vi "HFRR ADV v020 new software.vi"() -> ()   [LabVIEW 2025] (continued)
        n903 = call "File Dialog"("start path"=path "C:/LAB-IQ/images", "error in"=w1078) -> ("selected path"=w1067:path, "error out"=w1076:errorcluster)  [unwired: 10 in, 2 out]
        "Image path  2" <- w1067
        n904 = call <vilib>:"Clear Errors.vi"("error in (no error)"=w1076) -> ("error out"=w1075:errorcluster)  [unwired: 5 in, 1 out]
        n905 = call "IMAGE ANALYSIS.vi"("Enum"=POST_ANALYSIS_ENUM."OPEN FILE", "error in"=w1075, "File Path"=w1067) -> ("error out"=w1074:errorcluster)  [unwired: 7 in, 1 out]
        n906 = call <vilib>:"Clear Errors.vi"("error in (no error)"=w1074) -> ("error out"=w1073:errorcluster)  [unwired: 5 in, 1 out]
        n907 = call "IMAGE ANALYSIS.vi"("Enum"=POST_ANALYSIS_ENUM."SHOW UI", "error in"=w1073) -> ("error out"=w1071:errorcluster)  [unwired: 8 in, 1 out]
        n908 = local write "Zoom Factore"(100.0 ("Zoom Factore")) -> ()
      }
    }
    n909 = case shown="True" w762 {
      selector: w762 -> [_ w1050]
      tunnel: w754 -> [w1047 w1055]
      tunnel: [w1047 w1049] -> _
      frame False {
      }
      frame True {
        n910 = Not(x=w1050) -> (.not. x?=w1048:bool)
        n911 = local read "Zoom Factore"() -> (w1053:dbl)
        n912 = local write "OUT"(w1048) -> ()
        n913 = call "IMAGE ANALYSIS.vi"("Enum"=POST_ANALYSIS_ENUM."ZOOM OUT", "error in"=w1055) -> ("error out"=w1049:errorcluster)  [unwired: 8 in, 1 out]
        n914 = Divide(x=w1053, y=1.2) -> (x/y=w1051:dbl)
        n915 = local write "Zoom Factore"(w1051) -> ()
      }
    }
    n916 = case shown="True" w763 {
      selector: w763 -> [_ w1059]
      tunnel: w754 -> [w1056 w1064]
      tunnel: [w1056 w1057] -> _
      frame False {
      }
      frame True {
        n917 = Not(x=w1059) -> (.not. x?=w1058:bool)
        n918 = local read "Zoom Factore"() -> (w1062:dbl)
        n919 = local write "In"(w1058) -> ()
        n920 = call "IMAGE ANALYSIS.vi"("Enum"=POST_ANALYSIS_ENUM."ZOOM IN", "error in"=w1064) -> ("error out"=w1057:errorcluster)  [unwired: 8 in, 1 out]
        n921 = Multiply(x=w1062, y=1.2) -> (x*y=w1060:dbl)
        n922 = local write "Zoom Factore"(w1060) -> ()
      }
    }
    n923 = case shown="True" w759 {
      selector: w759 -> [_ w1031]
      tunnel: w754 -> [w1029 w1033]
      tunnel: [w1029 w1032] -> _
      frame False {
      }
      frame True {
        n924 = Not(x=w1031) -> (.not. x?=w1030:bool)
        n925 = local write "Clear ROI Tool"(w1030) -> ()
        n926 = call "IMAGE ANALYSIS.vi"("Enum"=POST_ANALYSIS_ENUM."CLEAR ROI", "error in"=w1033) -> ("error out"=w1032:errorcluster)  [unwired: 8 in, 1 out]
      }
    }
    n927 = case shown="True" w761 {
      selector: w761 -> [_ w1043]
      tunnel: w754 -> [w1041 w1046]
      tunnel: [w1041 w1044] -> _
      frame False {
      }
      frame True {
        n928 = Not(x=w1043) -> (.not. x?=w1042:bool)
        n929 = local write "line tool"(w1042) -> ()
        n930 = call "IMAGE ANALYSIS.vi"("Enum"=POST_ANALYSIS_ENUM."DRAW LINE", "error in"=w1046) -> ("error out"=w1044:errorcluster)  [unwired: 8 in, 1 out]
      }
    }
    n931 = case shown="True" w760 {
      selector: w760 -> [_ w1037]
      tunnel: w754 -> [w1035 w1039]
      tunnel: [w1035 w1038] -> _
      frame False {
      }
      frame True {
        n932 = Not(x=w1037) -> (.not. x?=w1036:bool)
        n933 = local write "Rectangle Tool"(w1036) -> ()
        n934 = call "IMAGE ANALYSIS.vi"("Enum"=POST_ANALYSIS_ENUM."DRAW REC", "error in"=w1039) -> ("error out"=w1038:errorcluster)  [unwired: 8 in, 1 out]
      }
    }
    n935 = local read "SCAR MEASURMENT"() -> (w747:enum32{"Auto Scar", "Manual Scar"})
    n936 = local read "Fit to Screen Tool"() -> (w756:bool)
    n937 = local read "Resize Tool"() -> (w755:bool)
    n938 = case shown="\"Manual Scar\", Default" w747 {
      frame "Auto Scar" {
        n939 = property on="Cap Live Image" class="Bool (strict)"("BoolText.Text"="Report" ("Boolean Text.Text")) -> ()  [unwired: 2 in, 2 out]
      }
      frame "Manual Scar", Default {
        n940 = property on="Cap Live Image" class="Bool (strict)"("BoolText.Text"="Save Image" ("Boolean Text.Text")) -> ()  [unwired: 2 in, 2 out]
      }
    }
    n941 = local read "ROI Color Tool"() -> (w757:bool)
    n942 = local read "Pan Tool"() -> (w758:bool)
    n943 = case shown="True" w758 {
      selector: w758 -> [_ w1025]
      tunnel: w754 -> [w1023 w1027]
      tunnel: [w1023 w1026] -> _
      frame False {
      }
      frame True {
        n944 = Not(x=w1025) -> (.not. x?=w1024:bool)
        n945 = call "IMAGE ANALYSIS.vi"("Enum"=POST_ANALYSIS_ENUM."PAN", "error in"=w1027) -> ("error out"=w1026:errorcluster)  [unwired: 8 in, 1 out]
        n946 = local write "Pan Tool"(w1024) -> ()
      }
    }
    n947 = case shown="True" w755 {
      selector: w755 -> [_ w1009]
      tunnel: w754 -> [w1004 w1006]
      tunnel: [w1004 w1005] -> _
      frame False {
      }
      frame True {
        n948 = Not(x=w1009) -> (.not. x?=w1008:bool)
        n949 = local write "Resize Tool"(w1008) -> ()
        n950 = call "IMAGE ANALYSIS.vi"("Enum"=POST_ANALYSIS_ENUM."RESIZE MODE", "error in"=w1006) -> ("error out"=w1005:errorcluster)  [unwired: 8 in, 1 out]
      }
    }
    n951 = case shown="True" w756 {
      selector: w756 -> [_ w1014]
      tunnel: [w1010 w1015] -> _
      tunnel: w754 -> [w1010 w1013]
      frame False {
      }
      frame True {
        n952 = Not(x=w1014) -> (.not. x?=w1012:bool)
        n953 = local write "Zoom Factore"(100.0 ("Zoom Factore")) -> ()
        n954 = local write "Fit to Screen Tool"(w1012) -> ()
        n955 = call "IMAGE ANALYSIS.vi"("Enum"=POST_ANALYSIS_ENUM."FIT", "error in"=w1013) -> ("error out"=w1015:errorcluster)  [unwired: 8 in, 1 out]
      }
    }
    n956 = case shown="True" w757 {
      selector: w757 -> [_ w1020]
      tunnel: [w1017 w1021] -> _
      tunnel: w754 -> [w1017 w1018]
      frame False {
      }
      frame True {
        n957 = Not(x=w1020) -> (.not. x?=w1019:bool)
        n958 = local write "ROI Color Tool"(w1019) -> ()
        n959 = call "IMAGE ANALYSIS.vi"("Enum"=POST_ANALYSIS_ENUM."SET ROI COLOR", "error in"=w1018) -> ("error out"=w1021:errorcluster)  [unwired: 8 in, 1 out]
      }
    }
    n960 = local read "Quit"() -> (w771:bool)
  }
  n961 = while {
    stop <- w1105 stop-if-true
    n962 = local read "Image Path"() -> (w1108:path)
    n963 = local read "Print 3"() -> (w1111:bool)
    n964 = Equal?(x=w1108, y=path "") -> (x = y?=w1107:bool)
    n965 = Not(x=w1107) -> (.not. x?=w1106:bool)
    n966 = property on="Print 3" class="Bool (strict)"("Visible"=w1106) -> ()  [unwired: 2 in, 2 out]
    n967 = case shown="True" w1111 {
      frame False {
        n968 = local write "Rd"(TRUE ("Boolean 7")) -> ()
      }
      frame True {
        n969 = flat-sequence {
          tunnel: [w1151] -> w1119
          tunnel: [w1138] -> w1117
          tunnel: [w1148] -> w1113
          tunnel: w1119 -> [w1160]
          tunnel: [w1160] -> w1118
          tunnel: w1117 -> [w1159]
          tunnel: [w1159] -> w1116
          tunnel: [w1157] -> w1115
          tunnel: [w1156] -> w1114
          tunnel: w1113 -> [w1156]
          tunnel: w1118 -> [w1162]
          tunnel: w1116 -> [w1163]
          tunnel: w1115 -> [_]
          tunnel: w1114 -> [w1161]
          frame #0 {
            n970 = case shown="True" "Rd" {
              frame False {
              }
              frame True {
                n971 = while {
                  tunnel: "abcdefABCDEF" ("string 2") -> [w1130]
                  shift-right: [w1128] -> w1122
                  shift-left: "" -> [w1127]
                  i -> [w1137]
                  stop <- w1136 stop-if-true
                  n972 = Random Number (0-1)() -> (number: 0 to 1=w1131:dbl)
                  n973 = Multiply(x=w1131, y=62.0) -> (x*y=w1133:dbl)
                  n974 = Decrement(x="Length 2") -> (x-1=w1126:i16)
                  n975 = To Word Integer(number=w1133) -> (16bit integer=w1134:i16)
                  n976 = String Subset(string=w1130, offset (0)=w1134, length (rest)=1 ("length (rest)")) -> (substring=w1129:string)
                  n977 = Greater Or Equal?(x=w1137, y=w1126) -> (x >= y?=w1136:bool)
                  n978 = Concatenate Strings(w1129, w1127) -> (w1128:string)
                }
                "String 10" <- w1122
                n979 = local write "Rd"(FALSE ("Boolean 7")) -> ()
              }
            }
          }
          frame #1 {
            w1149 = "_resized.jpg" ("command line")
            (unwired) ".jpg -resize 320x240 " ("string")
            (unwired) "Choose an Image File" ("prompt")
            # "-resize 1798x425"
            n980 = local read "Image Path"() -> (w1143:path)
            n981 = Strip Path(path=w1143) -> (stripped path=w1138:path, name=w1139:string)
            n982 = Match Pattern(string=w1139, regular expression=".jpg") -> (before substring=→"before substring 2":string, after substring=→"after substring":string)  [unwired: 1 in, 2 out]
            n983 = Match Pattern(string=w1139, regular expression="\\") -> (before substring=w1145:string)  [unwired: 1 in, 3 out]
            n984 = Match Pattern(string=w1145, regular expression=".jpg") -> (before substring=w1144:string)  [unwired: 1 in, 3 out]
            n985 = Concatenate Strings("cmd /c convert " ("string"), w1144, ".jpg -resize 320x240  " ("command line"), w1144, w1149) -> (w1152:string)
            n986 = call <vilib>:"System Exec.vi"("run minimized? (F)"=TRUE, "wait until completion? (T)"=TRUE, "working directory"=w1138, "command line"=w1152) -> ("error out"=w1151:errorcluster)  [unwired: 4 in, 3 out]
            "error out 2" <- w1151
            n987 = Concatenate Strings(w1144, w1149) -> (w1148:string)
          }
          frame #2 {
            n988 = Wait (ms)(milliseconds to wait=u32 2000 ("millisecond timer value")) -> (millisecond timer value=w1157:u32)
          }
          frame #3 {
            n989 = case shown="No Error" w1162 {
              tunnel: w1163 -> [w1166 _]
              tunnel: w1161 -> [w1164 _]
              frame No Error {
                (unwired) ".jpg" ("string")
                n990 = Path To String(path=w1166) -> (string=w1170:string)
                n991 = Concatenate Strings(w1170, "\\" ("string"), w1164) -> (w1169:string)
                n992 = String To Path(string=w1169) -> (path=w1168:path)
                n993 = call <vilib>:"Read JPEG File.vi"("path to JPEG file"=w1168) -> ("image data"=w1172:T16)  [unwired: 8 in, 2 out]
                "image data" <- w1172
                n994 = local write "Print 3"(FALSE ("Print 2")) -> ()
                n995 = call <vilib>:"Draw Flattened Pixmap.vi"("image data"=w1172) -> ("new picture"=→"new picture":picture)  [unwired: 8 in]
              }
              frame Error {
              }
            }
          }
        }
      }
    }
    n996 = Wait (ms)(milliseconds to wait=u32 20 ("millisecond timer value")) -> ()  [unwired: 1 out]
    n997 = local read "Quit"() -> (w1105:bool)
  }
  n998 = while {
    tunnel: w39 -> [_]
    tunnel: w23 -> [_]
    stop <- w1203 stop-if-true
    # "New Adv Logics"
    n999 = local read "Main Tab"() -> (w1183:T2)
    n1000 = local read "Main Tab"() -> (w1201:T2)
    n1001 = local read "Sign In"() -> (w1200:bool)
    n1002 = case shown="\"Adv Scar\"" w1183 {
      frame "HOME", Default {
        n1003 = local read "LIVE FEED MIN TEMP"() -> (w1336:bool)
        n1004 = local write "LIVE FEED MAX TEMP"(TRUE ("LIVE FEED MAX TEMP")) -> ()
        n1005 = local read "CAMERA ROI MIN TEMP"() -> (w1334:bool)
        n1006 = case shown="True" w1336 {
          selector: w1336 -> [_ w1343]
          frame False {
          }
          frame True {
            n1007 = Not(x=w1343) -> (.not. x?=w1342:bool)
            n1008 = local write "LIVE FEED MIN TEMP"(w1342) -> ()
            n1009 = call "CAMERA LIVE FEED FGV.vi"("Enum - Menu"=CAMERA_LIVE_FEED_ENUM."CAMERA MINIMIZE") -> ()  [unwired: 9 in, 2 out]
          }
        }
        n1010 = case shown="True" w1334 {
          selector: w1334 -> [_ w1340]
          frame False {
          }
          frame True {
            n1011 = Not(x=w1340) -> (.not. x?=w1339:bool)
            n1012 = local write "CAMERA ROI MIN TEMP"(w1339) -> ()
            n1013 = call "IMAGE ANALYSIS.vi"("Enum"=POST_ANALYSIS_ENUM."MINIMIZE UI") -> ()  [unwired: 9 in, 2 out]
          }
        }
        n1014 = local write "CAMERA ROI MAX TEMP"(TRUE ("CAMERA ROI MAX TEMP")) -> ()
      }
      frame "Test Setup" {
        n1015 = local read "LIVE FEED MIN TEMP"() -> (w1346:bool)
        n1016 = local read "CAMERA ROI MIN TEMP"() -> (w1344:bool)
        n1017 = local write "LIVE FEED MAX TEMP"(TRUE ("LIVE FEED MAX TEMP")) -> ()
        n1018 = case shown="True" w1346 {
          selector: w1346 -> [_ w1353]
          frame False {
          }
          frame True {
            n1019 = Not(x=w1353) -> (.not. x?=w1352:bool)
            n1020 = local write "LIVE FEED MIN TEMP"(w1352) -> ()
            n1021 = call "CAMERA LIVE FEED FGV.vi"("Enum - Menu"=CAMERA_LIVE_FEED_ENUM."CAMERA MINIMIZE") -> ()  [unwired: 9 in, 2 out]
          }
        }
        n1022 = case shown="True" w1344 {
          selector: w1344 -> [_ w1350]
          frame False {
          }
          frame True {
            n1023 = Not(x=w1350) -> (.not. x?=w1349:bool)
            n1024 = local write "CAMERA ROI MIN TEMP"(w1349) -> ()
            n1025 = call "IMAGE ANALYSIS.vi"("Enum"=POST_ANALYSIS_ENUM."MINIMIZE UI") -> ()  [unwired: 9 in, 2 out]
          }
        }
        n1026 = local write "CAMERA ROI MAX TEMP"(TRUE ("CAMERA ROI MAX TEMP")) -> ()
      }
      frame "Acquire" {
        n1027 = local read "LIVE FEED MIN TEMP"() -> (w1356:bool)
        n1028 = local write "LIVE FEED MAX TEMP"(TRUE ("LIVE FEED MAX TEMP")) -> ()
        n1029 = local read "CAMERA ROI MIN TEMP"() -> (w1354:bool)
        n1030 = case shown="True" w1356 {
          selector: w1356 -> [_ w1363]
          frame False {
          }
          frame True {
            n1031 = Not(x=w1363) -> (.not. x?=w1362:bool)
            n1032 = local write "LIVE FEED MIN TEMP"(w1362) -> ()
            n1033 = call "CAMERA LIVE FEED FGV.vi"("Enum - Menu"=CAMERA_LIVE_FEED_ENUM."CAMERA MINIMIZE") -> ()  [unwired: 9 in, 2 out]
          }
        }
        n1034 = case shown="True" w1354 {
          selector: w1354 -> [_ w1360]
          frame False {
          }
          frame True {
            n1035 = Not(x=w1360) -> (.not. x?=w1359:bool)
            n1036 = local write "CAMERA ROI MIN TEMP"(w1359) -> ()
            n1037 = call "IMAGE ANALYSIS.vi"("Enum"=POST_ANALYSIS_ENUM."MINIMIZE UI") -> ()  [unwired: 9 in, 2 out]
          }
        }
        n1038 = local write "CAMERA ROI MAX TEMP"(TRUE ("CAMERA ROI MAX TEMP")) -> ()
      }
      frame "Adv Scar" {
        n1039 = local read "CAMERA ROI MIN TEMP"() -> (w1364:bool)
        n1040 = case shown="True" "LIVE FEED MAX TEMP" {
          selector: "LIVE FEED MAX TEMP" -> [_ w1385]
          frame False {
          }
          frame True {
            n1041 = Not(x=w1385) -> (.not. x?=w1384:bool)
            n1042 = local write "LIVE FEED MAX TEMP"(w1384) -> ()
            n1043 = call "CAMERA LIVE FEED FGV.vi"("Enum - Menu"=CAMERA_LIVE_FEED_ENUM."CAMERA RESTORE") -> ("error out"=w1375:errorcluster)  [unwired: 9 in, 1 out]
            n1044 = Type Cast(type=30, x=0) -> (*(type *) &x=w1379:i32)
            n1045 = Add(x=w1379, y=48) -> (x+y=w1380:i32)
            n1046 = call "CAMERA LIVE FEED FGV.vi"("Enum - Menu"=CAMERA_LIVE_FEED_ENUM."CAMERA MODE SET", "error in (no error)"=w1375, "CAMERA MODE"=w1380) -> ("error out"=w1372:errorcluster)  [unwired: 7 in, 1 out]
            n1047 = call "CAMERA LIVE FEED FGV.vi"("Enum - Menu"=CAMERA_LIVE_FEED_ENUM."CAMERA GRAY", "error in (no error)"=w1372) -> ("error out"=w1371:errorcluster)  [unwired: 8 in, 1 out]
            n1048 = call "LIST FILE NAMES.vi"("error in (no error)"=w1371) -> ("error out"=w1381:errorcluster, "filenames"=w1382:string[])  [unwired: 9 in]
            n1049 = property on="FILE 3" class="CmbBox"(error in=w1381, "Strings[]"=w1382) -> ()  [unwired: 1 in, 2 out]
          }
        }
        n1050 = case shown="True" w1364 {
          selector: w1364 -> [_ w1370]
          frame False {
          }
          frame True {
            n1051 = Not(x=w1370) -> (.not. x?=w1369:bool)
            n1052 = local write "CAMERA ROI MIN TEMP"(w1369) -> ()
            n1053 = call "IMAGE ANALYSIS.vi"("Enum"=POST_ANALYSIS_ENUM."MINIMIZE UI") -> ()  [unwired: 9 in, 2 out]
          }
        }
        n1054 = local write "CAMERA ROI MAX TEMP"(TRUE ("CAMERA ROI MAX TEMP")) -> ()
        "LIVE FEED MIN TEMP" <- TRUE ("LIVE FEED MIN TEMP")
      }
      frame "Adv Scar Report" {
        n1055 = local read "CAMERA ROI MAX TEMP"() -> (w1386:bool)
        n1056 = local read "LIVE FEED MIN TEMP"() -> (w1388:bool)
        n1057 = local write "LIVE FEED MAX TEMP"(TRUE ("LIVE FEED MAX TEMP")) -> ()
        n1058 = case shown="True" w1388 {
          selector: w1388 -> [_ w1397]
          frame False {
          }
          frame True {
            n1059 = Not(x=w1397) -> (.not. x?=w1396:bool)
            n1060 = local write "LIVE FEED MIN TEMP"(w1396) -> ()
            n1061 = call "CAMERA LIVE FEED FGV.vi"("Enum - Menu"=CAMERA_LIVE_FEED_ENUM."CAMERA MINIMIZE") -> ()  [unwired: 9 in, 2 out]
          }
        }
        n1062 = case shown="True" w1386 {
          selector: w1386 -> [_ w1394]
          frame False {
          }
          frame True {
            n1063 = Not(x=w1394) -> (.not. x?=w1392:bool)
            n1064 = local write "CAMERA ROI MAX TEMP"(w1392) -> ()
            n1065 = call "IMAGE ANALYSIS.vi"("Enum"=POST_ANALYSIS_ENUM."SHOW UI") -> ("error out"=w1391:errorcluster)  [unwired: 9 in, 1 out]
            n1066 = call "LIST FILE NAMES.vi"("error in (no error)"=w1391) -> ("filenames"=w1390:string[])  [unwired: 9 in, 1 out]
            n1067 = property on="Test File List :" class="CmbBox"("Strings[]"=w1390) -> ()  [unwired: 2 in, 2 out]
          }
        }
        n1068 = local write "CAMERA ROI MIN TEMP"(TRUE ("CAMERA ROI MIN TEMP")) -> ()
      }
      frame "Compare Files" {
        n1069 = local read "LIVE FEED MIN TEMP"() -> (w1400:bool)
        n1070 = local write "LIVE FEED MAX TEMP"(TRUE ("LIVE FEED MAX TEMP")) -> ()
        n1071 = local read "CAMERA ROI MIN TEMP"() -> (w1398:bool)
        n1072 = case shown="True" w1400 {
          selector: w1400 -> [_ w1407]
          frame False {
          }
          frame True {
            n1073 = Not(x=w1407) -> (.not. x?=w1406:bool)
            n1074 = local write "LIVE FEED MIN TEMP"(w1406) -> ()
            n1075 = call "CAMERA LIVE FEED FGV.vi"("Enum - Menu"=CAMERA_LIVE_FEED_ENUM."CAMERA MINIMIZE") -> ()  [unwired: 9 in, 2 out]
          }
        }
        n1076 = case shown="True" w1398 {
          selector: w1398 -> [_ w1404]
          frame False {
          }
          frame True {
            n1077 = Not(x=w1404) -> (.not. x?=w1403:bool)
            n1078 = local write "CAMERA ROI MIN TEMP"(w1403) -> ()
            n1079 = call "IMAGE ANALYSIS.vi"("Enum"=POST_ANALYSIS_ENUM."MINIMIZE UI") -> ()  [unwired: 9 in, 2 out]
          }
        }
        n1080 = local write "CAMERA ROI MAX TEMP"(TRUE ("CAMERA ROI MAX TEMP")) -> ()
      }
      frame "About" {
        n1081 = local read "LIVE FEED MIN TEMP"() -> (w1410:bool)
        n1082 = local write "LIVE FEED MAX TEMP"(TRUE ("LIVE FEED MAX TEMP")) -> ()
        n1083 = local read "CAMERA ROI MIN TEMP"() -> (w1409:bool)
        n1084 = case shown="True" w1410 {
          selector: w1410 -> [_ w1417]
          frame False {
          }
          frame True {
            n1085 = Not(x=w1417) -> (.not. x?=w1416:bool)
            n1086 = local write "LIVE FEED MIN TEMP"(w1416) -> ()
            n1087 = call "CAMERA LIVE FEED FGV.vi"("Enum - Menu"=CAMERA_LIVE_FEED_ENUM."CAMERA MINIMIZE") -> ()  [unwired: 9 in, 2 out]
          }
        }
        n1088 = case shown="True" w1409 {
          selector: w1409 -> [_ w1414]
          frame False {
          }
          frame True {
            n1089 = Not(x=w1414) -> (.not. x?=w1413:bool)
            n1090 = local write "CAMERA ROI MIN TEMP"(w1413) -> ()
            n1091 = call "IMAGE ANALYSIS.vi"("Enum"=POST_ANALYSIS_ENUM."MINIMIZE UI") -> ()  [unwired: 9 in, 2 out]
          }
        }
        n1092 = local write "CAMERA ROI MAX TEMP"(TRUE ("CAMERA ROI MIN TEMP")) -> ()
      }
      frame "Advance" {
        n1093 = local read "LIVE FEED MIN TEMP"() -> (w1420:bool)
        n1094 = local write "LIVE FEED MAX TEMP"(TRUE ("LIVE FEED MAX TEMP")) -> ()
        n1095 = local read "CAMERA ROI MIN TEMP"() -> (w1418:bool)
        n1096 = case shown="True" w1420 {
          selector: w1420 -> [_ w1427]
          frame False {
          }
          frame True {
            n1097 = Not(x=w1427) -> (.not. x?=w1426:bool)
            n1098 = local write "LIVE FEED MIN TEMP"(w1426) -> ()
            n1099 = call "CAMERA LIVE FEED FGV.vi"("Enum - Menu"=CAMERA_LIVE_FEED_ENUM."CAMERA MINIMIZE") -> ()  [unwired: 9 in, 2 out]
          }
        }
        n1100 = local write "CAMERA ROI MAX TEMP"(TRUE ("CAMERA ROI MAX TEMP")) -> ()
        n1101 = case shown="True" w1418 {
          selector: w1418 -> [_ w1424]
          frame False {
          }
          frame True {
            n1102 = Not(x=w1424) -> (.not. x?=w1423:bool)
            n1103 = local write "CAMERA ROI MIN TEMP"(w1423) -> ()
            n1104 = call "IMAGE ANALYSIS.vi"("Enum"=POST_ANALYSIS_ENUM."MINIMIZE UI") -> ()  [unwired: 9 in, 2 out]
          }
        }
      }
      frame "Mooha" {
        n1105 = local read "LIVE FEED MIN TEMP"() -> (w1430:bool)
        n1106 = local write "LIVE FEED MAX TEMP"(TRUE ("LIVE FEED MAX TEMP")) -> ()
        n1107 = local read "CAMERA ROI MIN TEMP"() -> (w1428:bool)
        n1108 = case shown="True" w1430 {
          selector: w1430 -> [_ w1437]
          frame False {
          }
          frame True {
            n1109 = Not(x=w1437) -> (.not. x?=w1436:bool)
            n1110 = local write "LIVE FEED MIN TEMP"(w1436) -> ()
            n1111 = call "CAMERA LIVE FEED FGV.vi"("Enum - Menu"=CAMERA_LIVE_FEED_ENUM."CAMERA MINIMIZE") -> ()  [unwired: 9 in, 2 out]
          }
        }
        n1112 = local write "CAMERA ROI MAX TEMP"(TRUE ("CAMERA ROI MAX TEMP")) -> ()
        n1113 = case shown="True" w1428 {
          selector: w1428 -> [_ w1434]
          frame False {
          }
          frame True {
            n1114 = Not(x=w1434) -> (.not. x?=w1433:bool)
            n1115 = local write "CAMERA ROI MIN TEMP"(w1433) -> ()
            n1116 = call "IMAGE ANALYSIS.vi"("Enum"=POST_ANALYSIS_ENUM."MINIMIZE UI") -> ()  [unwired: 9 in, 2 out]
          }
        }
      }
    }
    n1117 = local read "Auto Start Test"() -> (w1174:bool)
    n1118 = case shown="True" "sign in temp" {
      frame False {
      }
      frame True {
        w1210 = 1 ("y")
        n1119 = local read "USERNAME"() -> (w1216:string)
        n1120 = local read "USER ID"() -> (w1213:string)
        n1121 = call <vilib>:"Trim Whitespace.vi"("string"=w1216) -> ("trimmed string"=w1215:string)  [unwired: 1 in]
        n1122 = call <vilib>:"Trim Whitespace.vi"("string"=w1213) -> ("trimmed string"=w1214:string)  [unwired: 1 in]
        n1123 = String Length(string=w1215) -> (length=w1212:i32)
        n1124 = String Length(string=w1214) -> (length=w1211:i32)
        n1125 = Greater?(x=w1212, y=w1210) -> (0:w1209:bool)
        n1126 = Greater?(x=w1211, y=w1210) -> (0:w1208:bool)
        n1127 = And(x=w1209, y=w1208) -> (x .and. y?=w1207:bool)
        n1128 = case shown="True" w1207 {
          frame False {
            n1129 = property on="Sign In" class="Bool (strict)"("DisabledEnum"=T19."Disabled" ("Disabled")) -> ()  [unwired: 2 in, 2 out]
          }
          frame True {
            n1130 = property on="Sign In" class="Bool (strict)"("DisabledEnum"=T19."Enabled" ("Disabled")) -> ()  [unwired: 2 in, 2 out]
          }
        }
      }
    }
    n1131 = local read "Air Temperature"() -> (w1191:bool)
    n1132 = local read "Coefficient Of Friction"() -> (w1192:bool)
    n1133 = case shown="False" w1174 {
      frame False {
        n1134 = local read "Auto stop temp"() -> (w1204:bool)
        n1135 = case shown="True" w1204 {
          frame False {
          }
          frame True {
            n1136 = local write "Auto Start Temp"(FALSE ("Auto Start Temp")) -> ()
          }
        }
      }
      frame True {
        "Auto stop temp" <- TRUE ("Auto stop temp")
      }
    }
    n1137 = local read "Humidity"() -> (w1190:bool)
    n1138 = case shown="\"HOME\"" w1201 {
      frame "HOME" {
        n1139 = local write "main tab sub"(enum32{"Page 1", "Page 2"}."Page 1" ("main tab sub")) -> ()
      }
      frame Default {
        n1140 = local write "main tab sub"(enum32{"Page 1", "Page 2"}."Page 2" ("main tab sub")) -> ()
      }
    }
    n1141 = case shown="True" w1200 {
      selector: w1200 -> [_ w1551]
      frame False {
      }
      frame True {
        n1142 = Not(x=w1551) -> (.not. x?=w1550:bool)
        n1143 = local write "Sign In"(w1550) -> ()
        n1144 = local write "Main Dashboard Buttons"(T24."Test Setup" ("Main Dashboard Buttons")) -> ()
      }
    }
    n1145 = case shown="\"Numeric Display\", Default" "Num/Graph" {
      frame "Numeric Display", Default {
        n1146 = property on="Single/Multiple" class="RadioBtnsControl (strict)"("Visible"=FALSE) -> ()  [unwired: 2 in, 2 out]
        n1147 = property on="Single - Graph" class="Ring (strict)"("Visible"=FALSE) -> ()  [unwired: 2 in, 2 out]
        n1148 = local write "Main Tab Display"(T4."Dashboard 1" ("Main Tab Display")) -> ()
      }
      frame "Graph Display" {
        n1149 = property on="Single/Multiple" class="RadioBtnsControl (strict)"("Visible"=TRUE) -> ()  [unwired: 2 in, 2 out]
        n1150 = case shown="\"Multiple\"" "Single/Multiple" {
          frame "Single ", Default {
            n1151 = property on="Single - Graph" class="Ring (strict)"("Visible"=TRUE) -> ()  [unwired: 2 in, 2 out]
            n1152 = local write "Main Tab Display"(T4."Dashboard 3" ("Main Tab Display")) -> ()
          }
          frame "Multiple" {
            n1153 = property on="Single - Graph" class="Ring (strict)"("Visible"=FALSE) -> ()  [unwired: 2 in, 2 out]
            n1154 = local write "Main Tab Display"(T4."Dashboard 2" ("Main Tab Display")) -> ()
          }
        }
      }
    }
    n1155 = local read "Stroke"() -> (w1189:bool)
    n1156 = local read "USERNAME"() -> (w1195:string)
    n1157 = local read "USER ID"() -> (w1194:string)
    n1158 = case shown="True" w1192 {
      selector: w1192 -> [_ w1477]
      frame False {
      }
      frame True {
        n1159 = Not(x=w1477) -> (.not. x?=w1476:bool)
        n1160 = local write "Coefficient Of Friction"(w1476) -> ()
        n1161 = local write "Tab Control 2"(T6."Coefficient Of Friction" ("Tab Control 2")) -> ()
      }
    }
    n1162 = case shown="True" w1191 {
      selector: w1191 -> [_ w1474]
      frame False {
      }
      frame True {
        n1163 = Not(x=w1474) -> (.not. x?=w1472:bool)
        n1164 = local write "Air Temperature"(w1472) -> ()
        n1165 = local write "Tab Control 2"(T6."Air Temperature" ("Tab Control 2")) -> ()
      }
    }
    n1166 = local write "Operator ID"(w1194) -> ()
    n1167 = case shown="True" w1189 {
      selector: w1189 -> [_ w1468]
      frame False {
      }
      frame True {
        n1168 = Not(x=w1468) -> (.not. x?=w1466:bool)
        n1169 = local write "Stroke"(w1466) -> ()
        n1170 = local write "Tab Control 2"(T6."Stroke" ("Tab Control 2")) -> ()
      }
    }
    n1171 = local write "tested by"(w1195) -> ()
    n1172 = case shown="True" w1190 {
      selector: w1190 -> [_ w1471]
      frame False {
      }
      frame True {
        n1173 = Not(x=w1471) -> (.not. x?=w1469:bool)
        n1174 = local write "Humidity"(w1469) -> ()
        n1175 = local write "Tab Control 2"(T6."Humidity" ("Tab Control 2")) -> ()
      }
    }
    n1176 = case shown="\"Calibration\"" "Main Dashboard Buttons" {
      tunnel: [T2."HOME" ("Main Tab") T2."Test Setup" ("Main Tab") T2."Acquire" ("Main Tab") T2."Adv Scar" ("Main Tab") T2."Adv Scar Report" ("Main Tab") T2."Compare Files" ("Main Tab") T2."Calibration" ("Main Tab") T2."About" ("Main Tab") T2."Advance" ("Main Tab")] -> w1173
      frame "Home", Default {
      }
      frame "Test Setup" {
      }
      frame "Dashboard" {
      }
      frame "Imaging" {
      }
      frame "Report" {
      }
      frame "Analysis" {
      }
      frame "Calibration" {
      }
      frame "About" {
      }
      frame "Advance" {
      }
    }
    n1177 = Wait (ms)(milliseconds to wait=u32 100) -> ()  [unwired: 1 out]
    n1178 = local read "Main Tab Display"() -> (w1193:T4)
    n1179 = local write "Main Tab"(w1173) -> ()
    n1180 = case shown="\"Dashboard 3\"" w1193 {
      frame "Dashboard 1", Default {
        n1181 = property on="Reset Graph" class="Bool (strict)"("Visible"=FALSE) -> ()  [unwired: 2 in, 2 out]
      }
      frame "Dashboard 2" {
        n1182 = property on="Reset Graph" class="Bool (strict)"("Visible"=TRUE) -> ()  [unwired: 2 in, 2 out]
      }
      frame "Dashboard 3" {
        n1183 = property on="Reset Graph" class="Bool (strict)"("Visible"=TRUE) -> ()  [unwired: 2 in, 2 out]
      }
    }
    n1184 = local read "SCAR MEASURMENT"() -> (w1181:enum32{"Auto Scar", "Manual Scar"})
    n1185 = local read "Humidity"() -> (w1196:bool)
    n1186 = local read "Cap Live Image"() -> (w1178:bool)
    n1187 = local read "Sample Temperature"() -> (w1188:bool)
    n1188 = local read "Air Temp vs Humidity"() -> (w1186:bool)
    n1189 = local read "Frequency"() -> (w1187:bool)
    n1190 = case shown="True" w1196 {
      frame False {
        n1191 = local write "Humidity On Command"(TRUE ("Humidity On Command")) -> ()
        n1192 = case shown="True" "Humidity Off Command" {
          selector: "Humidity Off Command" -> [_ w1484]
          frame False {
          }
          frame True {
            n1193 = stacked-sequence {
              frame #0 {
                n1194 = local read "WriteHumidity 2"() -> (w1486:string[])
                n1195 = Insert Into Array(array=w1486, new element="R;1" ("new element/subarray")) -> (w1485:string[])  [unwired: 1 in]
                n1196 = local write "WriteHumidity 2"(w1485) -> ()
              }
              frame #1 {
                n1197 = Wait (ms)(milliseconds to wait=u32 2000) -> ()  [unwired: 1 out]
              }
              frame #2 {
                n1198 = local read "WriteHumidity 2"() -> (w1489:string[])
                n1199 = local read "EVENT LOG"() -> (w1493:string)
                n1200 = call "Event Log.vi"("Content"="Humidity Control Off" ("string"), "EVENT LOG"=w1493) -> ("EVENT LOG"=w1494:string)  [unwired: 8 in, 1 out]
                n1201 = local write "EVENT LOG"(w1494) -> ()
                n1202 = Insert Into Array(array=w1489, new element="R;1" ("new element/subarray")) -> (w1490:string[])  [unwired: 1 in]
                n1203 = local write "WriteHumidity 2"(w1490) -> ()
              }
            }
            n1204 = Not(x=w1484) -> (.not. x?=w1483:bool)
            n1205 = local write "Humidity Off Command"(w1483) -> ()
          }
        }
      }
      frame True {
        n1206 = local write "Humidity Off Command"(TRUE ("Humidity Off Command")) -> ()
        n1207 = case shown="True" "Humidity On Command" {
          selector: "Humidity On Command" -> [_ w1498]
          frame False {
          }
          frame True {
            n1208 = stacked-sequence {
              frame #0 {
                n1209 = local read "Set Rh"() -> (w1504:dbl)
                n1210 = local read "WriteHumidity 2"() -> (w1499:string[])
                n1211 = Number To Fractional String(number=w1504, precision (6)=i16 2) -> (F-format string=w1505:string)  [unwired: 2 in]
                n1212 = Concatenate Strings("M;" ("new element/subarray"), w1505) -> (w1503:string)
                n1213 = Insert Into Array(array=w1499, new element=w1503) -> (w1500:string[])  [unwired: 1 in]
                n1214 = local write "WriteHumidity 2"(w1500) -> ()
              }
              frame #1 {
                n1215 = Wait (ms)(milliseconds to wait=u32 2000) -> ()  [unwired: 1 out]
              }
              frame #2 {
                n1216 = local read "Set Rh"() -> (w1512:dbl)
                n1217 = local read "WriteHumidity 2"() -> (w1507:string[])
                n1218 = Number To Fractional String(number=w1512, precision (6)=i16 2) -> (F-format string=w1513:string)  [unwired: 2 in]
                n1219 = Concatenate Strings("M;" ("new element/subarray"), w1513) -> (w1511:string)
                n1220 = Insert Into Array(array=w1507, new element=w1511) -> (w1508:string[])  [unwired: 1 in]
                n1221 = local write "WriteHumidity 2"(w1508) -> ()
              }
              frame #3 {
                n1222 = Wait (ms)(milliseconds to wait=u32 1500) -> ()  [unwired: 1 out]
              }
              frame #4 {
                (unwired) "% RH" ("string")
                (unwired) i16 2 ("precision (6)")
                (unwired) "M;" ("new element/subarray")
                n1223 = local read "Set Rh"() -> (w1522:dbl)
                n1224 = local read "WriteHumidity 2"() -> (w1515:string[])
                n1225 = Number To Fractional String(number=w1522, precision (6)=i16 2) -> (F-format string=w1519:string)  [unwired: 2 in]
                n1226 = Concatenate Strings("M;" ("new element/subarray"), w1519) -> (w1523:string)
                n1227 = Concatenate Strings("Humidity Set to : " ("string"), w1519, "% RH" ("string")) -> (w1517:string)
                n1228 = Insert Into Array(array=w1515, new element=w1523) -> (w1516:string[])  [unwired: 1 in]
                n1229 = disable-structure shown="Enabled" {
                  frame Enabled {
                    n1230 = local read "EVENT LOG"() -> (w1526:string)
                    n1231 = call "Event Log.vi"("Content"="Humidity Control On", "EVENT LOG"=w1526) -> ("EVENT LOG"=w1527:string)  [unwired: 8 in, 1 out]
                    n1232 = local write "EVENT LOG"(w1527) -> ()
                  }
                  frame Disabled {
                  }
                }
                n1233 = disable-structure shown="Enabled" {
                  disable-tunnel: w1517 -> [_ _]
                  frame Enabled {
                    n1234 = local read "EVENT LOG"() -> (w1529:string)
                    n1235 = call "Event Log.vi"("Content"="Humidity Control On", "EVENT LOG"=w1529) -> ("EVENT LOG"=w1530:string)  [unwired: 8 in, 1 out]
                    n1236 = local write "EVENT LOG"(w1530) -> ()
                  }
                  frame Disabled {
                  }
                }
                n1237 = local write "WriteHumidity 2"(w1516) -> ()
              }
            }
            n1238 = Not(x=w1498) -> (.not. x?=w1497:bool)
            n1239 = local write "Humidity On Command"(w1497) -> ()
          }
        }
      }
    }
    n1240 = Equal?(x=w1181, y=enum32{"Auto Scar", "Manual Scar"}."Auto Scar" ("SCAR MEASURMENT")) -> (x = y?=w1177:bool)
    n1241 = local read "TEST STANDARD"() -> (w1184:T3)
    n1242 = And(x=w1178, y=w1177) -> (x .and. y?=w1179:bool)
    n1243 = case shown="True" w1179 {
      selector: w1179 -> [_ w1283]
      tunnel: errorcluster {"status"=FALSE, "code"=0, "source"=""} ("error in (no error) 3") -> [_ w1284]
      frame False {
      }
      frame True {
        n1244 = stacked-sequence {
          tunnel: w1284 -> [_ _ _ _ _ _ _ w1332]
          tunnel: w1283 -> [_ _ _ _ _ w1313 _ _]
          frame #0 {
            n1245 = call "CAMERA LIVE FEED FGV.vi"("Enum - Menu"=CAMERA_LIVE_FEED_ENUM."CAMERA MINIMIZE") -> ()  [unwired: 9 in, 2 out]
          }
          frame #1 {
            n1246 = property on="Auto Scar Check  2" class="Clust (strict)"("Visible"=TRUE) -> ()  [unwired: 2 in, 2 out]
          }
          frame #2 {
            n1247 = String To Path(string="C:\\LAB-IQ\\Image Calibrate v01.dcf") -> (path=w1289:path)
            n1248 = Open/Create/Replace File ("Open File")(file path (use dialog)=w1289) -> (refnum out=w1290:refnum<file>)  [unwired: 5 in, 2 out]
            n1249 = for {
              N: 4 -> [_]
              tunnel: w1290 -> [w1296]
              i -> [w1292]
              n1250 = Read from Text File ("Read File")(file (use dialog)=w1296) -> (text=w1297:string)  [unwired: 3 in, 3 out]
              n1251 = String Subset(string=w1297, offset (0)=6, length (rest)=10 ("length (rest)")) -> (substring=w1293:string)
              n1252 = Fract/Exp String To Number(string=w1293) -> (number=w1291:dbl)  [unwired: 3 in, 1 out]
              n1253 = case shown="0" w1292 {
                tunnel: w1291 -> [w1298 w1299 _ w1300 _]
                frame 0 {
                  "5x Gain" <- w1298
                }
                frame 1 {
                  "10x Gain" <- w1299
                }
                frame 2 {
                }
                frame 3 {
                  "100x gain" <- w1300
                }
                frame 4, Default {
                }
              }
            }
          }
          frame #3 {
            n1254 = local read "FILE 3"() -> (w1306:string)
            n1255 = call <vilib>:"Trim Whitespace.vi"("string"="C:\\LAB-IQ\\images\\") -> ("trimmed string"=w1308:string)  [unwired: 1 in]
            n1256 = String To Path(string=w1308) -> (path=w1307:path)
            n1257 = Concatenate Strings(w1306, ".png" ("string")) -> (w1305:string)
            n1258 = Build Path(base path=w1307, name or relative path=w1305) -> (appended path=w1303:path)
            "Image path" <- w1303
            n1259 = Path To String(path=w1303) -> (string=w1302:string)
            n1260 = call "CAMERA LIVE FEED FGV.vi"("Enum - Menu"=CAMERA_LIVE_FEED_ENUM."CAMERA SAVE", "Image Path"=w1302) -> ()  [unwired: 8 in, 2 out]
          }
          frame #4 {
            n1261 = One Button Dialog(message="Image saved successfully") -> ()  [unwired: 1 in, 1 out]
          }
          frame #5 {
            n1262 = local read "TEST STANDARD"() -> (w1312:T3)
            n1263 = local read "Magnification len live scar"() -> (w1324:string)
            n1264 = Not(x=w1313) -> (.not. x?=w1314:bool)
            n1265 = local write "Cap Live Image"(w1314) -> ()
            n1266 = case shown="\"ISO 12156\"" w1312 {
              tunnel: ["ASTM D6079" "ISO 12156"] -> w1311
              frame "ASTM D6079", Default {
              }
              frame "ISO 12156" {
              }
            }
            n1267 = case shown="\"5x\", Default" w1324 {
              tunnel: [w1327 w1328] -> w1323
              frame "5x", Default {
                n1268 = local read "5x Gain"() -> (w1327:dbl)
              }
              frame "10x" {
                # "5x"
                n1269 = local read "10x Gain"() -> (w1328:dbl)
              }
            }
            n1270 = local read "Image path"() -> (w1322:path)
            n1271 = local read "FILE 3"() -> (w1315:string)
            n1272 = call "EDGE DETCTION.vi"("GAIN VALUE"=w1323, "Image Path"=w1322) -> ("error out"=w1321:errorcluster, "return value"=w1320:cluster{string, string, dbl, dbl, dbl})  [unwired: 8 in]
            n1273 = Bundle By Name(cluster=T25 {"File Name"="", "Test Method"="", "Operator"="", "Fuel Description"="", "Date and time"=""} ("Main Ref"), "File Name"=w1315, "Test Method"=w1311) -> (w1316:T25)
            n1274 = call "duf file read.vi"("error in (no error)"=w1321, "Main Ref"=w1316) -> ("error out"=w1319:errorcluster, "Main Ref 2"=w1317:T25)  [unwired: 8 in]
            n1275 = call "EDGE DETECTION REPORT.vi"("error in (no error)"=w1319, "return value 2"=w1320, "Main Ref"=w1317) -> ()  [unwired: 8 in, 1 out]
          }
          frame #6 {
            n1276 = property on="Auto Scar Check  2" class="Clust (strict)"("Visible"=FALSE) -> ()  [unwired: 2 in, 2 out]
          }
          frame #7 {
            n1277 = call "CAMERA LIVE FEED FGV.vi"("Enum - Menu"=CAMERA_LIVE_FEED_ENUM."CAMERA MINIMIZE", "error in (no error)"=w1332) -> ()  [unwired: 8 in, 2 out]
            n1278 = local write "Main Dashboard Buttons"(T1."Home" ("Main Dashboard Buttons")) -> ()
            n1279 = local write "Main Tab"(T2."HOME" ("Main Tab")) -> ()
          }
        }
      }
    }
    n1280 = local read "Heater Button"() -> (w1185:bool)
    n1281 = case shown="True" w1187 {
      selector: w1187 -> [_ w1462]
      frame False {
      }
      frame True {
        n1282 = Not(x=w1462) -> (.not. x?=w1460:bool)
        n1283 = local write "Frequency"(w1460) -> ()
        n1284 = local write "Tab Control 2"(T6."Frequency" ("Tab Control 2")) -> ()
      }
    }
    n1285 = case shown="True" w1186 {
      selector: w1186 -> [_ w1459]
      frame False {
      }
      frame True {
        n1286 = Not(x=w1459) -> (.not. x?=w1457:bool)
        n1287 = local write "Air Temp vs Humidity"(w1457) -> ()
        n1288 = local write "Tab Control 2"(T6."Air Temp vs Rh" ("Tab Control 2")) -> ()
      }
    }
    n1289 = case shown="True" w1188 {
      selector: w1188 -> [_ w1465]
      frame False {
      }
      frame True {
        n1290 = Not(x=w1465) -> (.not. x?=w1463:bool)
        n1291 = local write "Sample Temperature"(w1463) -> ()
        n1292 = local write "Tab Control 2"(T6."Sample Temperature" ("Tab Control 2")) -> ()
      }
    }
    n1293 = case shown="\"Custom\"" w1184 {
      frame "ASTM D6079", Default {
        w1438 = "ASTM D6079 TEST CONDITIONS" ("Standard 2")
        n1294 = local write "Standard 2"(w1438) -> ()
        n1295 = local write "Standard"(w1438) -> ()
      }
      frame "ISO 12156" {
        w1439 = "ISO 12156 TEST CONDITIONS" ("Standard 2")
        n1296 = local write "Standard 2"(w1439) -> ()
        n1297 = local write "Standard"(w1439) -> ()
      }
      frame "CEC F-096-A-06" {
        w1440 = "CEC F-096-A-06 TEST CONDITIONS" ("Standard 2")
        n1298 = local write "Standard 2"(w1440) -> ()
        n1299 = local write "Standard"(w1440) -> ()
      }
      frame "Custom" {
        w1441 = "CUSTOM TEST CONDITIONS" ("Standard 2")
        n1300 = local write "Standard 2"(w1441) -> ()
        n1301 = local write "Standard"(w1441) -> ()
      }
    }
    n1302 = case shown="True" w1185 {
      frame False {
        n1303 = local write "Temperature On Command"(TRUE ("Temperature On Command")) -> ()
        n1304 = case shown="True" "Temperature Off Command" {
          selector: "Temperature Off Command" -> [_ w1445]
          frame False {
          }
          frame True {
            n1305 = Not(x=w1445) -> (.not. x?=w1444:bool)
            n1306 = local read "EVENT LOG"() -> (w1448:string)
            n1307 = local write "Temperature Off Command"(w1444) -> ()
            n1308 = call "Event Log.vi"("Content"="Heater Off", "EVENT LOG"=w1448) -> ("EVENT LOG"=w1447:string)  [unwired: 8 in, 1 out]
            n1309 = local write "EVENT LOG"(w1447) -> ()
          }
        }
      }
      frame True {
        n1310 = local write "Temperature Off Command"(TRUE ("Temperature Off Command")) -> ()
        n1311 = case shown="True" "Temperature On Command" {
          selector: "Temperature On Command" -> [_ w1452]
          frame False {
          }
          frame True {
            n1312 = Not(x=w1452) -> (.not. x?=w1451:bool)
            n1313 = local write "Temperature On Command"(w1451) -> ()
            n1314 = disable-structure shown="Enabled" {
              disable-tunnel: "Heater On" -> [w1454 _]
              frame Enabled {
                n1315 = local read "EVENT LOG"() -> (w1455:string)
                n1316 = call "Event Log.vi"("Content"=w1454, "EVENT LOG"=w1455) -> ("EVENT LOG"=w1456:string)  [unwired: 8 in, 1 out]
                n1317 = local write "EVENT LOG"(w1456) -> ()
              }
              frame Disabled {
              }
            }
          }
        }
      }
    }
    n1318 = local read "Main Tab"() -> (w1176:T2)
    n1319 = case shown="\"About\"" w1176 {
      frame "HOME", Default {
        w1219 = T19."Enabled" ("Disabled")
        n1320 = local read "Service Password enable"() -> (w1221:bool)
        n1321 = property on="Imaging" class="Bool (strict)"("DisabledEnum"=w1219) -> ()  [unwired: 2 in, 2 out]
        n1322 = property on="Dashboard" class="Bool (strict)"("DisabledEnum"=w1219) -> ()  [unwired: 2 in, 2 out]
        n1323 = property on="Test Setup" class="Bool (strict)"("DisabledEnum"=w1219) -> ()  [unwired: 2 in, 2 out]
        n1324 = property on="Analysis" class="Bool (strict)"("DisabledEnum"=w1219) -> ()  [unwired: 2 in, 2 out]
        n1325 = property on="Home" class="Bool (strict)"("DisabledEnum"=w1219) -> ()  [unwired: 2 in, 2 out]
        n1326 = property on="Report" class="Bool (strict)"("DisabledEnum"=w1219) -> ()  [unwired: 2 in, 2 out]
        n1327 = property on="Main Dashboard Buttons" class="RadioBtnsControl (strict)"("DisabledEnum"=w1219) -> ()  [unwired: 2 in, 2 out]
        n1328 = property on="Calibration" class="Bool (strict)"("DisabledEnum"=w1219) -> ()  [unwired: 2 in, 2 out]
        n1329 = case shown="True" w1221 {
          tunnel: [T19."Disabled" ("Disabled") T19."Enabled" ("Disabled")] -> w1220
          frame False {
          }
          frame True {
          }
        }
        n1330 = property on="About" class="Bool (strict)"("DisabledEnum"=w1220) -> ()  [unwired: 2 in, 2 out]
      }
      frame "Test Setup" {
        w1226 = T19."Enabled" ("Disabled")
        n1331 = local read "Service Password enable"() -> (w1225:bool)
        n1332 = property on="Dashboard" class="Bool (strict)"("DisabledEnum"=T19."Disabled" ("Disabled")) -> ()  [unwired: 2 in, 2 out]
        n1333 = property on="Imaging" class="Bool (strict)"("DisabledEnum"=w1226) -> ()  [unwired: 2 in, 2 out]
        n1334 = property on="Analysis" class="Bool (strict)"("DisabledEnum"=w1226) -> ()  [unwired: 2 in, 2 out]
        n1335 = property on="Home" class="Bool (strict)"("DisabledEnum"=w1226) -> ()  [unwired: 2 in, 2 out]
        n1336 = property on="Report" class="Bool (strict)"("DisabledEnum"=w1226) -> ()  [unwired: 2 in, 2 out]
        n1337 = property on="Test Setup" class="Bool (strict)"("DisabledEnum"=w1226) -> ()  [unwired: 2 in, 2 out]
        n1338 = case shown="True" w1225 {
          tunnel: [T19."Disabled" ("Disabled") T19."Enabled" ("Disabled")] -> w1224
          frame False {
          }
          frame True {
          }
        }
        n1339 = property on="About" class="Bool (strict)"("DisabledEnum"=w1224) -> ()  [unwired: 2 in, 2 out]
      }
      frame "Adv Scar" {
        w1233 = T19."Enabled" ("Disabled")
        n1340 = property on="Dashboard" class="Bool (strict)"("DisabledEnum"=T19."Disabled" ("Disabled")) -> ()  [unwired: 2 in, 2 out]
        n1341 = property on="Imaging" class="Bool (strict)"("DisabledEnum"=w1233) -> ()  [unwired: 2 in, 2 out]
        n1342 = property on="Analysis" class="Bool (strict)"("DisabledEnum"=w1233) -> ()  [unwired: 2 in, 2 out]
        n1343 = property on="Home" class="Bool (strict)"("DisabledEnum"=w1233) -> ()  [unwired: 2 in, 2 out]
        n1344 = property on="Report" class="Bool (strict)"("DisabledEnum"=w1233) -> ()  [unwired: 2 in, 2 out]
        n1345 = property on="Test Setup" class="Bool (strict)"("DisabledEnum"=w1233) -> ()  [unwired: 2 in, 2 out]
        n1346 = local read "Service Password enable"() -> (w1231:bool)
        n1347 = case shown="True" w1231 {
          tunnel: [T19."Disabled" ("Disabled") T19."Enabled" ("Disabled")] -> w1230
          frame False {
          }
          frame True {
          }
        }
        n1348 = property on="About" class="Bool (strict)"("DisabledEnum"=w1230) -> ()  [unwired: 2 in, 2 out]
      }
      frame "Calibration" {
        w1236 = T19."Enabled" ("Disabled")
        n1349 = property on="Dashboard" class="Bool (strict)"("DisabledEnum"=T19."Disabled" ("Disabled")) -> ()  [unwired: 2 in, 2 out]
        n1350 = property on="Imaging" class="Bool (strict)"("DisabledEnum"=w1236) -> ()  [unwired: 2 in, 2 out]
        n1351 = property on="Analysis" class="Bool (strict)"("DisabledEnum"=w1236) -> ()  [unwired: 2 in, 2 out]
        n1352 = property on="Home" class="Bool (strict)"("DisabledEnum"=w1236) -> ()  [unwired: 2 in, 2 out]
        n1353 = property on="Report" class="Bool (strict)"("DisabledEnum"=w1236) -> ()  [unwired: 2 in, 2 out]
        n1354 = property on="Test Setup" class="Bool (strict)"("DisabledEnum"=w1236) -> ()  [unwired: 2 in, 2 out]
        n1355 = local read "Service Password enable"() -> (w1238:bool)
        n1356 = property on="Calibration" class="Bool (strict)"("DisabledEnum"=w1236) -> ()  [unwired: 2 in, 2 out]
        n1357 = case shown="True" w1238 {
          tunnel: [T19."Disabled" ("Disabled") T19."Enabled" ("Disabled")] -> w1237
          frame False {
          }
          frame True {
          }
        }
        n1358 = property on="About" class="Bool (strict)"("DisabledEnum"=w1237) -> ()  [unwired: 2 in, 2 out]
      }
      frame "Adv Scar Report" {
        w1244 = T19."Enabled" ("Disabled")
        n1359 = property on="Dashboard" class="Bool (strict)"("DisabledEnum"=T19."Disabled" ("Disabled")) -> ()  [unwired: 2 in, 2 out]
        n1360 = property on="Imaging" class="Bool (strict)"("DisabledEnum"=w1244) -> ()  [unwired: 2 in, 2 out]
        n1361 = property on="Analysis" class="Bool (strict)"("DisabledEnum"=w1244) -> ()  [unwired: 2 in, 2 out]
        n1362 = property on="Home" class="Bool (strict)"("DisabledEnum"=w1244) -> ()  [unwired: 2 in, 2 out]
        n1363 = property on="Report" class="Bool (strict)"("DisabledEnum"=w1244) -> ()  [unwired: 2 in, 2 out]
        n1364 = property on="Test Setup" class="Bool (strict)"("DisabledEnum"=w1244) -> ()  [unwired: 2 in, 2 out]
        n1365 = local read "Service Password enable"() -> (w1243:bool)
        n1366 = case shown="True" w1243 {
          tunnel: [T19."Disabled" ("Disabled") T19."Enabled" ("Disabled")] -> w1242
          frame False {
          }
          frame True {
          }
        }
        n1367 = property on="About" class="Bool (strict)"("DisabledEnum"=w1242) -> ()  [unwired: 2 in, 2 out]
      }
      frame "Compare Files" {
        w1250 = T19."Enabled" ("Disabled")
        n1368 = local read "Service Password enable"() -> (w1249:bool)
        n1369 = property on="Dashboard" class="Bool (strict)"("DisabledEnum"=T19."Disabled" ("Disabled")) -> ()  [unwired: 2 in, 2 out]
        n1370 = property on="Imaging" class="Bool (strict)"("DisabledEnum"=w1250) -> ()  [unwired: 2 in, 2 out]
        n1371 = property on="Analysis" class="Bool (strict)"("DisabledEnum"=w1250) -> ()  [unwired: 2 in, 2 out]
        n1372 = property on="Home" class="Bool (strict)"("DisabledEnum"=w1250) -> ()  [unwired: 2 in, 2 out]
        n1373 = property on="Report" class="Bool (strict)"("DisabledEnum"=w1250) -> ()  [unwired: 2 in, 2 out]
        n1374 = property on="Test Setup" class="Bool (strict)"("DisabledEnum"=w1250) -> ()  [unwired: 2 in, 2 out]
        n1375 = case shown="True" w1249 {
          tunnel: [T19."Disabled" ("Disabled") T19."Enabled" ("Disabled")] -> w1248
          frame False {
          }
          frame True {
          }
        }
        n1376 = property on="About" class="Bool (strict)"("DisabledEnum"=w1248) -> ()  [unwired: 2 in, 2 out]
      }
      frame "Acquire" {
        n1377 = local read "Service Password enable"() -> (w1255:bool)
        n1378 = property on="Test Setup" class="Bool (strict)"("DisabledEnum"=T19."Disabled" ("Disabled")) -> ()  [unwired: 2 in, 2 out]
        n1379 = local read "Auto Start Test"() -> (w1257:bool)
        n1380 = local read "RUN"() -> (w1259:bool)
        n1381 = case shown="True" w1255 {
          tunnel: [T19."Disabled" ("Disabled") T19."Enabled" ("Disabled")] -> w1256
          frame False {
          }
          frame True {
          }
        }
        n1382 = Or(x=w1259, y=w1257) -> (x .or. y?=w1258:bool)
        n1383 = case shown="True" w1258 {
          tunnel: [T19."Enabled" ("Disabled") T19."Disabled" ("Disabled")] -> w1254
          frame False {
          }
          frame True {
          }
        }
        n1384 = property on="About" class="Bool (strict)"("DisabledEnum"=w1256) -> ()  [unwired: 2 in, 2 out]
        n1385 = property on="Imaging" class="Bool (strict)"("DisabledEnum"=w1254) -> ()  [unwired: 2 in, 2 out]
        n1386 = property on="Dashboard" class="Bool (strict)"("DisabledEnum"=w1254) -> ()  [unwired: 2 in, 2 out]
        n1387 = property on="Analysis" class="Bool (strict)"("DisabledEnum"=w1254) -> ()  [unwired: 2 in, 2 out]
        n1388 = property on="Home" class="Bool (strict)"("DisabledEnum"=w1254) -> ()  [unwired: 2 in, 2 out]
        n1389 = property on="Report" class="Bool (strict)"("DisabledEnum"=w1254) -> ()  [unwired: 2 in, 2 out]
        n1390 = property on="Calibration" class="Bool (strict)"("DisabledEnum"=w1254) -> ()  [unwired: 2 in, 2 out]
      }
      frame "About" {
        n1391 = local read "FILE"() -> (w1273:string)
        n1392 = local read "TEST FILE NAM,E SAVED"() -> (w1266:bool)
        n1393 = call <vilib>:"Trim Whitespace.vi"("string"=w1273) -> ("trimmed string"=w1272:string)  [unwired: 1 in]
        n1394 = local read "Auto Start Test"() -> (w1276:bool)
        n1395 = String Length(string=w1272) -> (length=w1271:i32)
        n1396 = Greater?(x=w1271, y=1) -> (0:w1268:bool)
        n1397 = And(x=w1268, y=w1266) -> (x .and. y?=w1267:bool)
        n1398 = local read "RUN"() -> (w1278:bool)
        n1399 = case shown="True" w1267 {
          tunnel: [T19."Disabled" ("Disabled") T19."Enabled" ("Disabled")] -> w1269
          frame False {
          }
          frame True {
          }
        }
        n1400 = Or(x=w1278, y=w1276) -> (x .or. y?=w1277:bool)
        n1401 = property on="About" class="Bool (strict)"("DisabledEnum"=T19."Enabled" ("Disabled")) -> ()  [unwired: 2 in, 2 out]
        n1402 = case shown="False" w1277 {
          tunnel: [T19."Enabled" ("Disabled") T19."Disabled" ("Disabled")] -> w1275
          frame False {
          }
          frame True {
          }
        }
        n1403 = property on="Dashboard" class="Bool (strict)"("DisabledEnum"=w1269) -> ()  [unwired: 2 in, 2 out]
        n1404 = property on="Test Setup" class="Bool (strict)"("DisabledEnum"=T19."Disabled" ("Disabled")) -> ()  [unwired: 2 in, 2 out]
        n1405 = property on="Imaging" class="Bool (strict)"("DisabledEnum"=w1275) -> ()  [unwired: 2 in, 2 out]
        n1406 = property on="Analysis" class="Bool (strict)"("DisabledEnum"=w1275) -> ()  [unwired: 2 in, 2 out]
        n1407 = property on="Home" class="Bool (strict)"("DisabledEnum"=w1275) -> ()  [unwired: 2 in, 2 out]
        n1408 = property on="Report" class="Bool (strict)"("DisabledEnum"=w1275) -> ()  [unwired: 2 in, 2 out]
      }
    }
    n1409 = local read "Quit"() -> (w1203:bool)
    "Single" <- "Single - Graph"
  }
  n1410 = disable-structure shown="Disabled" {
    disable-tunnel: [w1555 _] -> w45
    disable-tunnel: _ -> [w1554 _]
    frame Disabled {
      n1411 = while {
        tunnel: w1554 -> [_]
        tunnel: [w1556] -> w1555
        tunnel: [w1557] -> _
        i -> [w1557]
        stop <- w1556 stop-if-true
        w1573 = u16 10 items=["1.0"=10, "1.5"=15, "2.0"=20] ("stop bits (10: 1 bit)")
        n1412 = Wait (ms)(milliseconds to wait=u32 10) -> ()  [unwired: 1 out]
        n1413 = call-poly "VISA Configure Serial Port"("VISA resource name"=refnum<visa-resource-name> "ASRL1::INSTR" ("COM PORT"), "timeout (10sec)"=u32 10, "baud rate (9600)"=u32 57600, "data bits (8)"=u16 8, "stop bits (10: 1 bit)"=w1573) -> ("VISA resource name out"=w1559:refnum<visa-resource-name>, "error out"=w1568:errorcluster)  [unwired: 9 in]
        n1414 = VISA Read(VISA resource name=w1559, byte count=u32 2 ("byte count (0)")) -> (read buffer=w1567:string)  [unwired: 1 in, 3 out]
        n1415 = String Subset(string=w1567, offset (0)=0, length (rest)=2 ("length (rest)")) -> (substring=w1566:string)
        n1416 = Match Pattern(string=w1566, regular expression="<>") -> (offset past match=w1563:i32)  [unwired: 1 in, 3 out]
        n1417 = Greater Or Equal?(x=w1563, y=0) -> (x >= y?=w1558:bool)
        n1418 = case shown="True" w1558 {
          tunnel: w1559 -> [_ w1577]
          tunnel: w1568 -> [_ w1576]
          frame False {
          }
          frame True {
            n1419 = VISA Read(VISA resource name=w1577, byte count=u32 32 ("byte count (0)"), error in (no error)=w1576) -> (read buffer=w1575:string)  [unwired: 3 out]
            n1420 = String Subset(string=w1575, offset (0)=0, length (rest)=8 ("length (rest)")) -> (substring=w1579:string)
            n1421 = String Subset(string=w1575, offset (0)=8, length (rest)=8 ("length (rest)")) -> (substring=w1580:string)
            n1422 = Decimal String To Number(string=w1580) -> (number=w1587:i32)  [unwired: 2 in, 1 out]
            n1423 = Decimal String To Number(string=w1579) -> (number=w1583:i32)  [unwired: 2 in, 1 out]
            n1424 = Divide(x=w1587, y=10000) -> ()  [unwired: 1 out]
            n1425 = Divide(x=w1583, y=1000000) -> ()  [unwired: 1 out]
          }
        }
        n1426 = local read "Quit"() -> (w1556:bool)
      }
    }
    frame Enabled {
    }
  }
  n1427 = Tick Count (ms)() -> (millisecond timer value=w2:u32)
  n1428 = while {
    shift-right: [w1627] -> _
    shift-left: w4 -> [w1631]
    shift-right: [w1626] -> _
    shift-left: w3 -> [w1630]
    shift-right: [w1625] -> _
    shift-left: w4 -> [w1629]
    shift-right: [w1624] -> _
    shift-left: w3 -> [w1628]
    shift-right: [w1622] -> _
    shift-left: w2 -> [w1623]
    shift-right: [w1619] -> _
    shift-left: w1 -> [w1620]
    shift-right: [w1618] -> _
    shift-left: w1 -> [w1621]
    shift-right: [w1611] -> _
    shift-left: w1 -> [w1617]
    shift-right: [w1610] -> _
    shift-left: w1 -> [w1616]
    shift-right: [w1609] -> _
    shift-left: w1 -> [w1615]
    shift-right: [w1608] -> _
    shift-left: w1 -> [w1614]
    shift-right: [w1607] -> _
    shift-left: w1 -> [w1613]
    shift-right: [w1606] -> _
    shift-left: w1 -> [w1612]
    shift-right: [w1605] -> _
    shift-left: w1 -> [w1599]
    shift-right: [w1604] -> _
    shift-left: w1 -> [w1598]
    shift-right: [w1603] -> _
    shift-left: w1 -> [w1597]
    shift-right: [w1602] -> _
    shift-left: w1 -> [w1596]
    shift-right: [w1601] -> _
    shift-left: w1 -> [w1595]
    shift-right: [w1600] -> _
    shift-left: w1 -> [w1594]
    stop <- w1634 stop-if-true
    n1429 = local read "Read Humidity"() -> (w1592:string)
    n1430 = local read "Error  2"() -> (w1632:errorcluster)
    n1431 = String Length(string=w1592) -> (length=w1591:i32)
    n1432 = call <vilib>:"Trim Whitespace.vi"("string"=w1592) -> ("trimmed string"=w1593:string)  [unwired: 1 in]
    n1433 = Greater Or Equal?(x=w1591, y=23) -> (x >= y?=w1589:bool)
    n1434 = case shown="No Error" w1632 {
      tunnel: w1631 -> [w1674 w1758]
      tunnel: w1630 -> [w1673 w1757]
      tunnel: w1629 -> [w1672 w1756]
      tunnel: w1628 -> [w1671 w1755]
      tunnel: [w1670 w1758] -> w1627
      tunnel: [w1669 w1757] -> w1626
      tunnel: [w1668 w1756] -> w1625
      tunnel: [w1667 w1755] -> w1624
      tunnel: w1623 -> [w1666 w1754]
      tunnel: [w1665 w1754] -> w1622
      tunnel: w1620 -> [w1664 w1753]
      tunnel: w1621 -> [w1663 w1752]
      tunnel: [w1662 w1753] -> w1619
      tunnel: [w1661 w1752] -> w1618
      tunnel: w1617 -> [w1660 w1751]
      tunnel: w1616 -> [w1659 w1750]
      tunnel: w1615 -> [w1658 w1749]
      tunnel: w1614 -> [w1657 w1748]
      tunnel: w1613 -> [w1656 w1747]
      tunnel: w1612 -> [w1655 w1746]
      tunnel: [w1654 w1751] -> w1611
      tunnel: [w1653 w1750] -> w1610
      tunnel: [w1652 w1749] -> w1609
      tunnel: [w1651 w1748] -> w1608
      tunnel: [w1650 w1747] -> w1607
      tunnel: [w1649 w1746] -> w1606
      tunnel: w1599 -> [w1648 w1745]
      tunnel: [w1647 w1745] -> w1605
      tunnel: [w1646 w1741] -> w1604
      tunnel: [w1645 w1740] -> w1603
      tunnel: [w1644 w1744] -> w1602
      tunnel: [w1643 w1743] -> w1601
      tunnel: [w1642 w1742] -> w1600
      tunnel: w1598 -> [w1641 w1744]
      tunnel: w1597 -> [w1640 w1743]
      tunnel: w1596 -> [w1639 w1742]
      tunnel: w1595 -> [w1638 w1741]
      tunnel: w1594 -> [w1637 w1740]
      tunnel: w1593 -> [w1636 _]
      tunnel: w1589 -> [w1635 _]
      frame No Error {
        n1435 = case shown="True" w1635 {
          tunnel: w1674 -> [w1687 w1733]
          tunnel: w1673 -> [w1686 w1732]
          tunnel: w1672 -> [w1685 w1731]
          tunnel: w1671 -> [w1684 w1730]
          tunnel: [w1687 w1729] -> w1670
          tunnel: [w1686 w1728] -> w1669
          tunnel: [w1685 w1727] -> w1668
          tunnel: [w1684 w1726] -> w1667
          tunnel: w1666 -> [w1683 w1724]
          tunnel: [w1683 w1723] -> w1665
          tunnel: w1664 -> [w1682 w1722]
          tunnel: w1663 -> [w1681 w1721]
          tunnel: [w1682 w1720] -> w1662
          tunnel: [w1681 w1719] -> w1661
          tunnel: w1660 -> [w1680 w1718]
          tunnel: w1659 -> [w1679 w1717]
          tunnel: w1658 -> [w1678 w1716]
          tunnel: w1657 -> [w1677 w1715]
          tunnel: w1656 -> [w1676 w1714]
          tunnel: w1655 -> [w1675 w1713]
          tunnel: [w1680 w1712] -> w1654
          tunnel: [w1679 w1711] -> w1653
          tunnel: [w1678 w1710] -> w1652
          tunnel: [w1677 w1709] -> w1651
          tunnel: [w1676 w1708] -> w1650
          tunnel: [w1675 w1707] -> w1649
          tunnel: w1648 -> [w1693 w1706]
          tunnel: [w1693 w1705] -> w1647
          tunnel: [w1690 w1704] -> w1646
          tunnel: [w1689 w1703] -> w1645
          tunnel: [w1692 w1702] -> w1644
          tunnel: [w1688 w1701] -> w1643
          tunnel: [w1691 w1700] -> w1642
          tunnel: w1641 -> [w1692 w1699]
          tunnel: w1640 -> [w1691 w1698]
          tunnel: w1639 -> [w1690 w1697]
          tunnel: w1638 -> [w1689 w1696]
          tunnel: w1637 -> [w1688 w1695]
          tunnel: w1636 -> [_ w1694]
          frame False {
          }
          frame True {
            n1436 = Tick Count (ms)() -> (millisecond timer value=w1725:u32)
            n1437 = String To Byte Array(string=w1694) -> (unsigned byte array=w1738:u8[])
            n1438 = Array Size(array=w1738) -> (size(s)=w1737:i32)
